vi "Menu Build Settings Item.vi"() -> (3 "Menu Settings Item":refnum<data-value>)   [LabVIEW 2018, in "Main Panel.lvlib" / "Main Panel.lvclass"]
uses:
  Main Panel.lvclass
  <userlib>/_MGI/Menu Building/MenuItem/MGI_MenuItem.lvclass
  Menu item.ctl
  <userlib>/_MGI/Menu Building/MenuItem/MenuItem.vi
  <userlib>/_MGI/Menu Building/MenuItem/Write Sub-Menus.vi
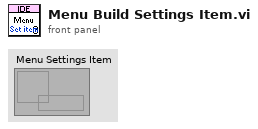
[diagram p1: front panel]
types:
  T1 = typedef "Main Panel.lvlib/Main Panel.lvclass/Menu Item.ctl" = enum16{"Invalid Item", "File", "Open File", "Save File", "Exit", "Settings", "Preferences", "Help", "Show Context Help"}
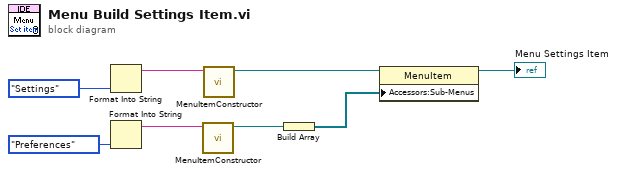
[diagram p0: block diagram]
diagram:
  n1 = Format Into String(Menu_Item."Settings" ("Menu item")) -> (resulting string=w1:string)  [unwired: 3 in, 1 out]
  n2 = Format Into String(Menu_Item."Preferences" ("Menu item")) -> (resulting string=w5:string)  [unwired: 3 in, 1 out]
  n3 = call-poly <userlib>:"MenuItemConstructor.vi"("Text"=w5) -> ("MenuItem"=w3:refnum<data-value>)  [unwired: 9 in, 1 out]
  n4 = call-poly <userlib>:"MenuItemConstructor.vi"("Text"=w1) -> ("MenuItem"=w8:refnum<data-value>)  [unwired: 9 in, 1 out]
  n5 = Build Array(w3) -> (w7:refnum<data-value>[])
  n6 = property class="MenuItem"(reference=w8, "Accessors:Sub-Menus"=w7) -> (reference out=→"Menu Settings Item":refnum<data-value>)  [unwired: 1 in, 1 out]
